vi "A0.vi"(4 "e^2":ext format="%.5g") -> (1 "A0":ext format="%.20g")   [LabVIEW 2015, in "Biblioteka moduł map v3.lvlib" / "Konwersja wsp.lvlib" / "UTM.lvlib" / "Konwersja z UTM na wsp geograficzne.lvlib"]
uses:
  Konwersja z UTM na wsp geograficzne.lvlib
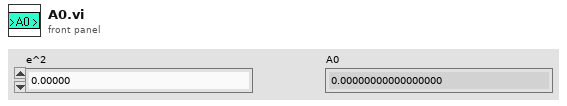
[diagram p1: front panel]
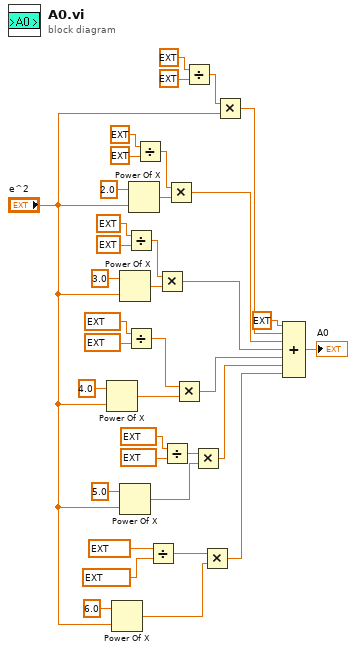
[diagram p0: block diagram]
diagram:
  n1 = Power Of X(1:"e^2", 2:4.0 ("y")) -> (0:w9:ext)
  n2 = Power Of X(1:"e^2", 2:6.0 ("y")) -> (0:w7:ext)
  n3 = Power Of X(1:"e^2", 2:3.0 ("y")) -> (0:w10:ext)
  n4 = Power Of X(1:"e^2", 2:5.0 ("y")) -> (0:w8:ext)
  n5 = Divide(x=ext 175.0, y=ext 256.0) -> (x/y=w29:ext)
  n6 = Divide(x=ext 11025.0, y=ext 16384.0) -> (x/y=w24:ext)
  n7 = Power Of X(1:"e^2", 2:2.0 ("y")) -> (0:w11:ext)
  n8 = Divide(x=ext 45.0, y=ext 64.0) -> (x/y=w30:ext)
  n9 = Divide(x=ext 693693.0, y=ext 1048576.0) -> (x/y=w18:ext)
  n10 = Multiply(x=w29, y=w10) -> (x*y=w16:ext)
  n11 = Divide(x=ext 43659.0, y=ext 65536.0) -> (x/y=w23:ext)
  n12 = Multiply(x=w30, y=w11) -> (x*y=w17:ext)
  n13 = Multiply(x=w24, y=w9) -> (x*y=w15:ext)
  n14 = Divide(x=ext 3.0, y=ext 4.0) -> (x/y=w36:ext)
  n15 = Multiply(x=w23, y=w8) -> (x*y=w14:ext)
  n16 = Multiply(x=w18, y=w7) -> (x*y=w13:ext)
  n17 = Multiply(x=w36, y="e^2") -> (x*y=w33:ext)
  n18 = Compound Arithmetic op=ADD(ext 1.0 ("x"), w33, w17, w16, w15, w14, w13) -> (→"A0":ext)
